vi "Send OVP.vi"(8 "error in (no error)":errorcluster, 11 "79XRP in":refnum<class "7976A.lvclass">) -> (0 "error out":errorcluster, 3 "79XRP out":refnum<class "7976A.lvclass">)   [LabVIEW 2019, in "7976A.lvlib" / "7976A.lvclass"]
uses:
  Library/7976A.lvclass
  C:/Users/Public/Documents/Development/builds/Instruments/PowerSupply.lvlibp/Library/PowerSupply.lvclass
  Library/7976A.lvclass/7976A.ctl
  builds/Engine/Engine.lvlibp/Project/Engine.lvclass
  <instrlib>/Agilent N7976A/Agilent N7976A.lvlib
  C:/Users/Public/Documents/Development/builds/Engine/Engine.lvlibp/Project/Engine.lvclass
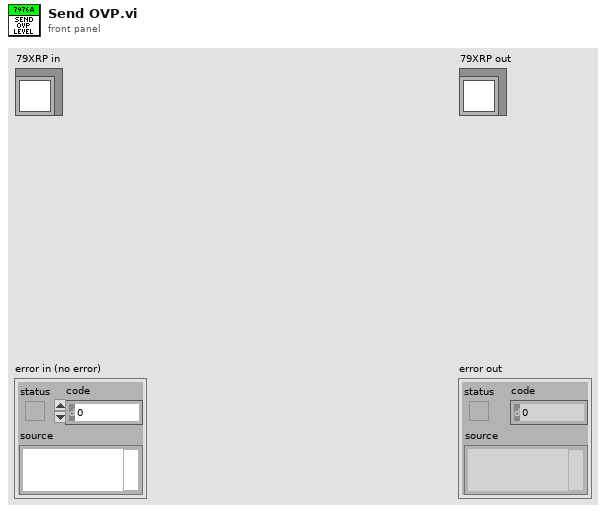
[diagram p1: front panel]
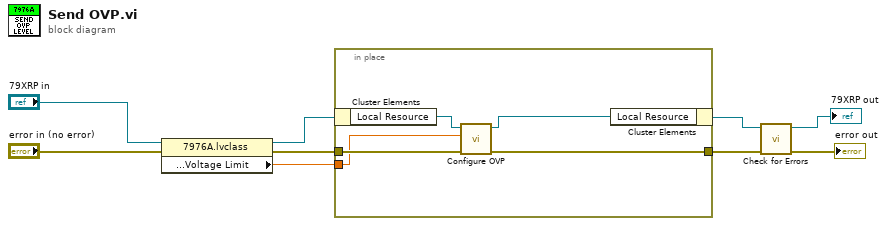
[diagram p0: block diagram]
diagram:
  n1 = property class="7976A.lvclass"(reference="79XRP in", error in="error in (no error)") -> (reference out=w5:refnum<class "7976A.lvclass">, error out=w3:errorcluster, "Accessors:Setting:Protection:Voltage Limit"=w1:dbl)
  n2 = in-place {
    in-place-border: w3 -> [w14]
    in-place-border: [w11] -> w2
    in-place-border: w1 -> [w10]
    n3 = in-place-cluster #1(w5) -> ("Local Resource"=w13:refnum<visa-resource-name>)
    n4 = call <instrlib>:"Configure OVP.vi"("error in (no error)"=w14, "OVP Protection (48V)"=w10, "VISA resource name"=w13) -> ("error out"=w11:errorcluster, "VISA resource name out"=w12:refnum<visa-resource-name>)  [unwired: 7 in]
    n5 = in-place-cluster #1("Local Resource"=w12) -> (w4:refnum<class "7976A.lvclass">)
  }
  n6 = call "Check for Errors.vi"("error in"=w2, "Engine in"=w4) -> ("error out"=→"error out":errorcluster, "Engine out"=→"79XRP out":refnum<class "7976A.lvclass">)  [unwired: 8 in]
